vi "Actor Core.vi"(8 "error in":errorcluster, 11 "CS++DMMGui.lvclass":refnum<class "CS++DMMGui.lvclass">) -> (0 "error out":errorcluster, 3 "Actor out":refnum<class "Actor.lvclass">)   [LabVIEW 2013, in "CS++DMMGui.lvlib" / "CS++DMMGui.lvclass"]
doc: "(<B>Filename</B>: Actor Framework.lvlib:Actor.lvclass:Actor Core.vi)\n\nReceives messages to the actor, reacts to them, and initiates any error handling that may shut the actor down.\n\nDescendant classes may override this VI to append parallel tasks for the actor to complete while it handles messages. Overrides use the Call Parent Method node."
uses:
  CS++DMMGui.lvclass
  <vilib>/ActorFramework/Actor/Actor.lvclass
  Core/Actors/CS++SVMonitor/CS++SVMonitor.lvclass
  CS++DMMGui Messages/UpdateReading/UpdateReading Msg.lvclass
  CS++DMMGui Messages/UpdateMPReading/UpdateMPReading Msg.lvclass
  Core/Actors/CS++BaseActor/CS++BaseActor.lvclass/CS++BaseActor.ctl
  <vilib>/ActorFramework/Actor/Actor.lvclass/Actor.ctl
  <vilib>/ActorFramework/Message Enqueuer/Message Enqueuer.lvclass/Message Enqueuer.ctl
  Core/Actors/CS++DeviceGUIActor/CS++DeviceGUIActor.lvclass/CS++DeviceGUIActor.ctl
  Core/Classes/CS++BaseClasses/Factory/CS++Factory.lvclass
  Core/Actors/CS++PVMonitor/CS++PVMonitor.lvclass/CS++PVMonitor.ctl
  Core/Actors/CS++GUIActor/CS++GUIActor.lvclass/CS++GUIActor.ctl
  CS++DMMGui.lvclass/CS++DMMGui.ctl
  Core/Actors/CS++PVMonitor Messages/Register PVs Msg/Register PVs Msg.lvclass/Register PVs Msg.ctl
  Core/Actors/CS++DeviceGUIActor/CS++DeviceGUIActor.lvclass
  CS++DMM Messages/Configure Measurement Msg/Configure Measurement Msg.lvclass/Configure Measurement Msg.ctl
  CS++DMM Messages/Configure AC Bandwidth [AC] Msg/Configure AC Bandwidth [AC] Msg.lvclass/Configure AC Bandwidth [AC] Msg.ctl
  CS++DMM Messages/Configure Frequency Voltage Range [FVR] Msg/Configure Frequency Voltage Range [FVR] Msg.lvclass/Configure Frequency Voltage Range [FVR] Msg.ctl
  CS++DMM Messages/Configure Tranducer Type [TMP] Msg/Configure Tranducer Type [TMP] Msg.lvclass/Configure Tranducer Type [TMP] Msg.ctl
  CS++DMM Messages/Configure Thermocouple [TC] Msg/Configure Thermocouple [TC] Msg.lvclass/Configure Thermocouple [TC] Msg.ctl
  CS++DMM Messages/Configure Fixed Ref Junction [TC] Msg/Configure Fixed Ref Junction [TC] Msg.lvclass/Configure Fixed Ref Junction [TC] Msg.ctl
  CS++DMM Messages/Configure RTD [RTD] Msg/Configure RTD [RTD] Msg.lvclass/Configure RTD [RTD] Msg.ctl
  CS++DMM Messages/Configure Thermistor [THM] Msg/Configure Thermistor [THM] Msg.lvclass/Configure Thermistor [THM] Msg.ctl
  CS++DMM Messages/Configure Trigger Msg/Configure Trigger Msg.lvclass/Configure Trigger Msg.ctl
  CS++DMM Messages/Configure Trigger Slope [TS] Msg/Configure Trigger Slope [TS] Msg.lvclass/Configure Trigger Slope [TS] Msg.ctl
  CS++DMM Messages/Configure Multi-Point [MP] Msg/Configure Multi-Point [MP] Msg.lvclass/Configure Multi-Point [MP] Msg.ctl
  CS++DMM Messages/Configure Meas Complete Dest [MP] Msg/Configure Meas Complete Dest [MP] Msg.lvclass/Configure Meas Complete Dest [MP] Msg.ctl
  CS++DMM Messages/Configure Auto Zero Mode [AZ] Msg/Configure Auto Zero Mode [AZ] Msg.lvclass/Configure Auto Zero Mode [AZ] Msg.ctl
  CS++DMM Messages/Configure Power Line Frequency [PLF] Msg/Configure Power Line Frequency [PLF] Msg.lvclass/Configure Power Line Frequency [PLF] Msg.ctl
  Core/Actors/CS++DeviceGUIActor/Read Resource Name.vi
  Core/Actors/CS++DeviceGUIActor/Read Driver Revision.vi
  Core/Actors/CS++DeviceGUIActor/Read Firmware Revision.vi
  Core/Actors/CS++DeviceGUIActor/Read Self-Test Result Code.vi
  Core/Actors/CS++DeviceGUIActor/Read Self-Test Result Message.vi
  <vilib>/ActorFramework/Message Enqueuer/Init from Existing Queue.vi
  <vilib>/ActorFramework/Message Enqueuer/Enqueue.vi
  <vilib>/ActorFramework/Message Priority Queue/Priority Enqueue.vi
  <vilib>/ActorFramework/Message Enqueuer/Message Enqueuer.lvclass
  Core/Actors/CS++PVMonitor Messages/Register PVs Msg/Register PVs Msg.lvclass
  <vilib>/ActorFramework/Stop Msg/Stop Msg.lvclass
  CS++DMM Messages/Configure Measurement Msg/Configure Measurement Msg.lvclass
  CS++DMM Messages/Configure AC Bandwidth [AC] Msg/Configure AC Bandwidth [AC] Msg.lvclass
  CS++DMM Messages/Configure Frequency Voltage Range [FVR] Msg/Configure Frequency Voltage Range [FVR] Msg.lvclass
  CS++DMM Messages/Configure Tranducer Type [TMP] Msg/Configure Tranducer Type [TMP] Msg.lvclass
  CS++DMM Messages/Configure Thermocouple [TC] Msg/Configure Thermocouple [TC] Msg.lvclass
  CS++DMM Messages/Configure Fixed Ref Junction [TC] Msg/Configure Fixed Ref Junction [TC] Msg.lvclass
  CS++DMM Messages/Configure RTD [RTD] Msg/Configure RTD [RTD] Msg.lvclass
  CS++DMM Messages/Configure Thermistor [THM] Msg/Configure Thermistor [THM] Msg.lvclass
  CS++DMM Messages/Configure Trigger Msg/Configure Trigger Msg.lvclass
  CS++DMM Messages/Configure Trigger Slope [TS] Msg/Configure Trigger Slope [TS] Msg.lvclass
  CS++DMM Messages/Configure Multi-Point [MP] Msg/Configure Multi-Point [MP] Msg.lvclass
  CS++DMM Messages/Configure Meas Complete Dest [MP] Msg/Configure Meas Complete Dest [MP] Msg.lvclass
  CS++DMM Messages/Configure Auto Zero Mode [AZ] Msg/Configure Auto Zero Mode [AZ] Msg.lvclass
  CS++DMM Messages/Configure Power Line Frequency [PLF] Msg/Configure Power Line Frequency [PLF] Msg.lvclass
  Core/Actors/CS++BaseActor/CS++BaseActor.lvclass
  Core/Actors/CS++GUIActor/CS++GUIActor.lvclass
  Core/Actors/CS++PVMonitor/CS++PVMonitor.lvclass
panel:
  in  "Tab Control":T1(tab)
  out "Actor Name":string
  out "Driver Revision":string
  out "Firmware Revision":string
  out "Self-Test Result Code":i32
  out "Self-Test Result Message":string
  out "Resource Name":string
  in  "Configuration Tab":T2(tab)
  in  "freq volt range (10.0 V RMS)":dbl=10.0 format="%^.2e"
  in  "ac max frequency (300.0E+3 Hz)":dbl=300000.0 format="%^.2e"
  in  "ac min frequency (20.0 Hz)":dbl=20.0 format="%^.2e"
  in  "range (-1.0: Auto)":dbl=-1.0 format="%^.2e"
  in  "measurement function (DC Volts)":i32(ring)=1 items=["DC Volts"=1, "AC Volts"=2, "DC Current"=3, "AC Current"=4, "2 Wire Resistance"=5, "4 Wire Resistance"=101, "AC + DC Volts"=106, "AC + DC Current"=107, "Frequency"=104, "Period"=105, "Temperature"=108]
  in  "auto zero mode (Off)":i32(ring) items=["On"=1, "Off"=0, "Once"=2]
  in  "power line frequency (50.0 Hz)":dbl=50.0 caption="power line frequency (60.0 Hz)" format="%^.2e"
  in  "Tranducer Tab":enum32{"Thermocouple", "RTD", "Thermistor"}(tab)
  in  "fixed ref junc (0.0 Celsius)":dbl format="%^.2e"
  in  "ref junc type (Internal)":i32(ring)=1 items=["Internal"=1, "Fixed"=2]
  in  "thermocouple type (B)":i32(ring)=1 items=["B"=1, "C"=2, "D"=3, "E"=4, "G"=5, "J"=6, "K"=7, "N"=8, "R"=9, "S"=10, "T"=11, "U"=12, "V"=13]
  in  "resistance (0.0 ohms)":dbl format="%^.2e"
  in  "alpha (0.0)":dbl format="%^.2e"
  in  "resistance (0.0 ohms)":dbl format="%^.2e"
  in  "transducer type (Thermocouple)":i32(ring)=1 items=["Thermocouple"=1, "Thermistor"=2, "2-Wire RTD"=3, "4-Wire RTD"=4]
  in  "trigger source (Immediate)":i32(ring)=1 items=["Immediate"=1, "External"=2, "Software Trigger Function"=3, "PXI TRIG0 or VXI TTL0"=111, "PXI TRIG1 or VXI TTL1"=112, "PXI TRIG2 or VXI TTL2"=113, "PXI TRIG3 or VXI TTL3"=114, "PXI TRIG4 or VXI TTL4"=115, "PXI TRIG5 or VXI TTL5"=116, "PXI TRIG6 or VXI TTL6"=117, "PXI TRIG7 or VXI TTL7"=118, "ECL0"=119, "ECL1"=120, "PXI Star"=131, "RTSI 0"=140, "RTSI 1"=141, "RTSI 2"=142, "RTSI 3"=143, "RTSI 4"=144, "RTSI 5"=145, "RTSI 6"=146]
  in  "trigger delay (0.0 s)":dbl format="%.3f"
  in  "trigger slope (0: Positive)":i32(ring) items=["Positive", "Negative"]
  in  "sample interval (0.0 s)":dbl format="%.3f"
  in  "sample trigger (Immediate)":i32(ring)=1 items=["Immediate"=1, "External"=2, "Software Trigger Function"=3, "Interval"=10, "PXI TRIG0 or VXI TTL0"=111, "PXI TRIG1 or VXI TTL1"=112, "PXI TRIG2 or VXI TTL2"=113, "PXI TRIG3 or VXI TTL3"=114, "PXI TRIG4 or VXI TTL4"=115, "PXI TRIG5 or VXI TTL5"=116, "PXI TRIG6 or VXI TTL6"=117, "PXI TRIG7 or VXI TTL7"=118, "ECL0"=119, "ECL1"=120, "PXI Star"=131, "RTSI 0"=140, "RTSI 1"=141, "RTSI 2"=142, "RTSI 3"=143, "RTSI 4"=144, "RTSI 5"=145, "RTSI 6"=146]
  in  "trigger count (1)":i32=1
  in  "sample count (1)":i32=1
  in  "meas complete dest (None)":i32(ring)=-1 items=["None"=-1, "External"=2, "PXI TRIG0 or VXI TTL0"=111, "PXI TRIG1 or VXI TTL1"=112, "PXI TRIG2 or VXI TTL2"=113, "PXI TRIG3 or VXI TTL3"=114, "PXI TRIG4 or VXI TTL4"=115, "PXI TRIG5 or VXI TTL5"=116, "PXI TRIG6 or VXI TTL6"=117, "PXI TRIG7 or VXI TTL7"=118, "ECL0"=119, "ECL1"=120, "PXI Star"=131, "RTSI 0"=140, "RTSI 1"=141, "RTSI 2"=142, "RTSI 3"=143, "RTSI 4"=144, "RTSI 5"=145, "RTSI 6"=146]
  out "Waveform Chart":dbl(graph)
  out "Waveform Graph":dbl[](graph)
  in  "Stop Button":bool
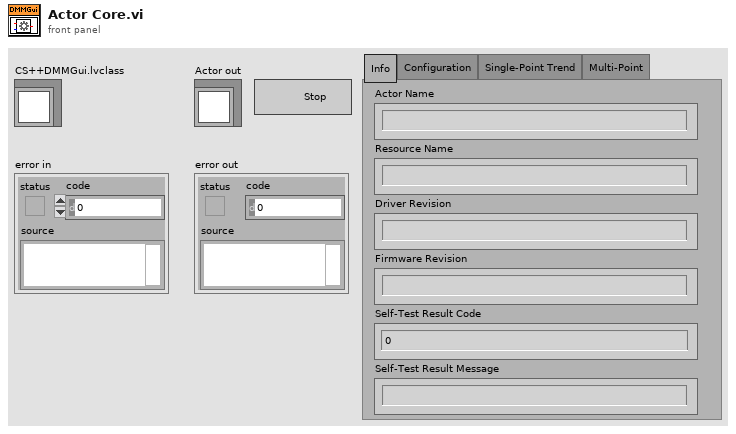
[diagram p1: front panel]
types:
  T1 = enum32{"Info", "Configuration", "Single-Point Trend", "Multi-Point"}
  T2 = enum32{"General", "Transducer", "Trigger", "Multi-Point"}
  T3 = enum32{"Invalid", "Standard", "Closed", "Hidden", "Minimized", "Maximized"}
  T4 = cluster{"name":string, "CS++DMMGui.lvlib:UpdateReading.lvclass":refnum<class "UpdateReading Msg.lvclass">}
  T5 = cluster{"name":string, "CS++DMMGui.lvlib:UpdateMPReading Msg.lvclass":refnum<class "UpdateMPReading Msg.lvclass">}
  T6 = cluster{"name":string, "CS++DMMGui.lvlib:UpdateMPReading Msg.lvclass":refnum<class "CS++PVUpdate Msg.lvclass">}[]
  T7 = cluster{"Self Enqueuer":refnum<class "Message Enqueuer.lvclass">, cluster{"name":string, "CS++DMMGui.lvlib:UpdateMPReading Msg.lvclass":refnum<class "CS++PVUpdate Msg.lvclass">}[]}
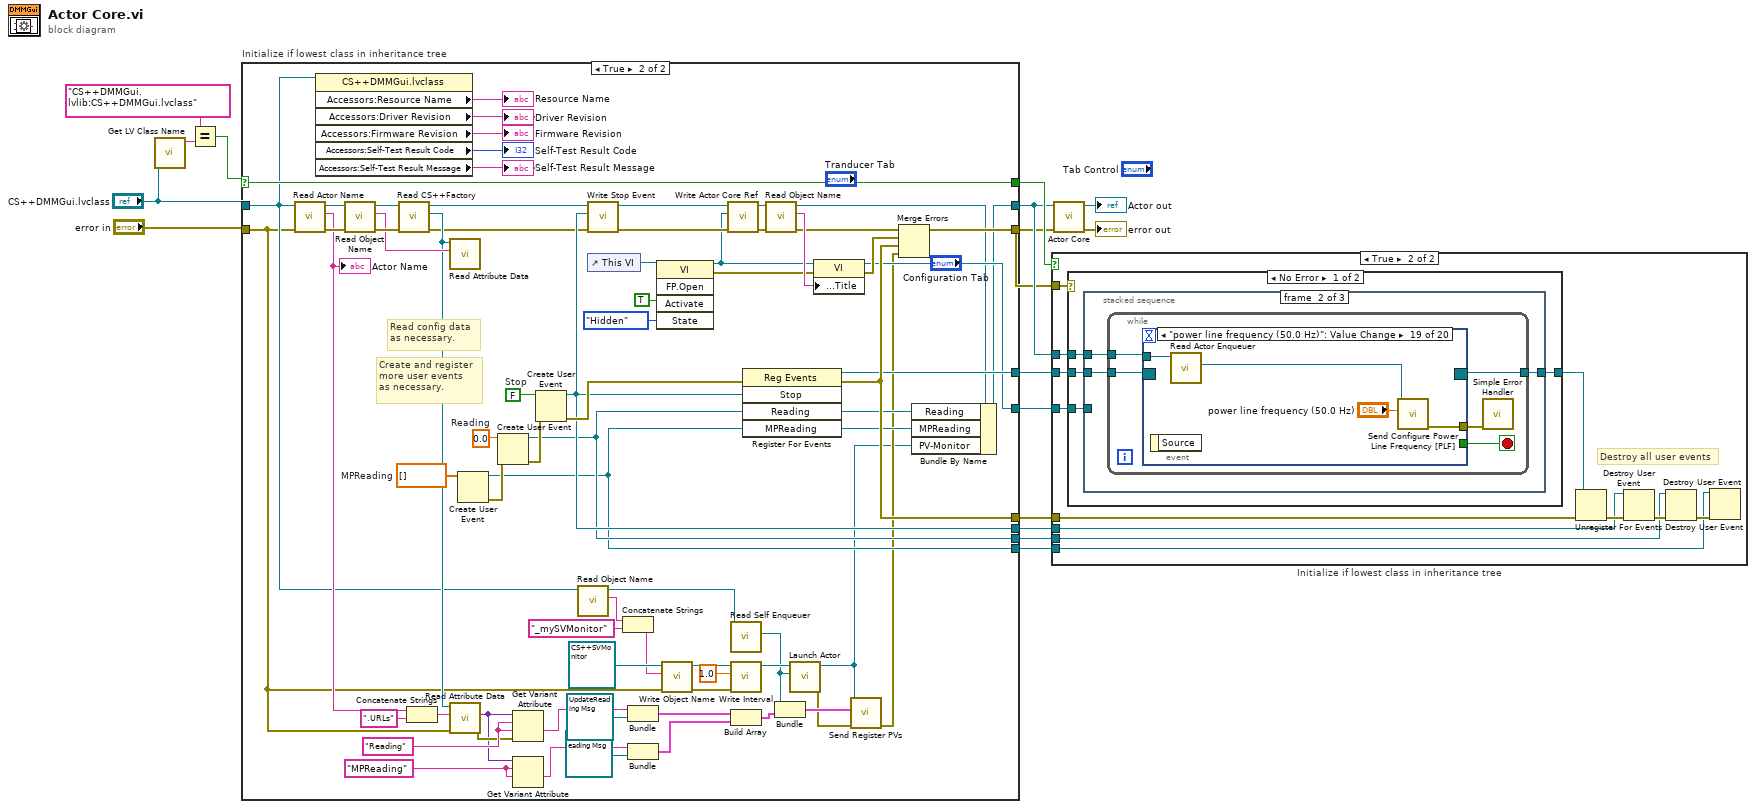
[diagram p0: block diagram]
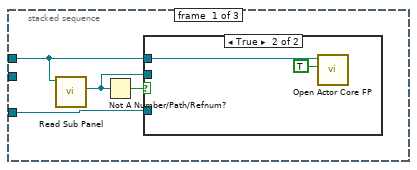
[diagram p4: hidden frame]
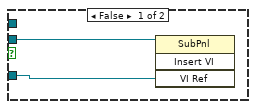
[diagram p5: hidden frame]
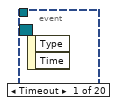
[diagram p6: hidden frame]
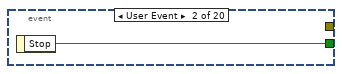
[diagram p7: hidden frame]
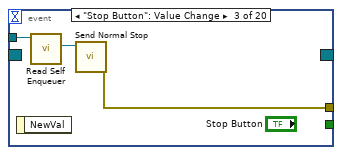
[diagram p8: hidden frame]
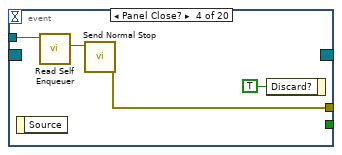
[diagram p9: hidden frame]
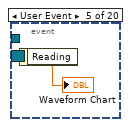
[diagram p10: hidden frame]
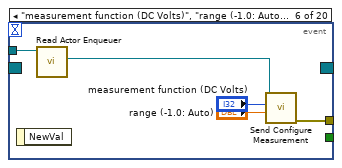
[diagram p11: hidden frame]
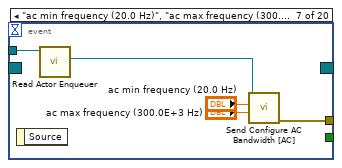
[diagram p12: hidden frame]
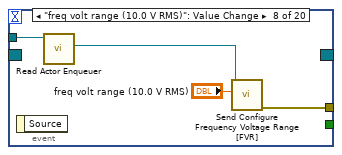
[diagram p13: hidden frame]
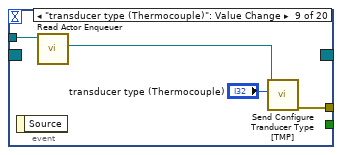
[diagram p14: hidden frame]
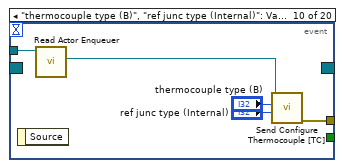
[diagram p15: hidden frame]
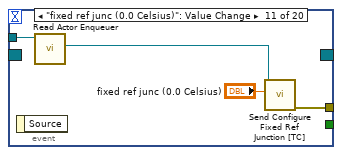
[diagram p16: hidden frame]
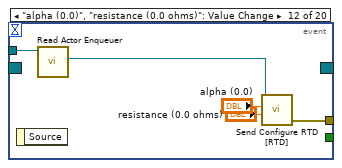
[diagram p17: hidden frame]
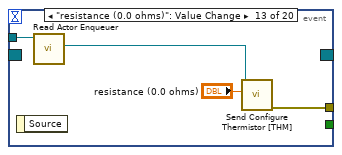
[diagram p18: hidden frame]
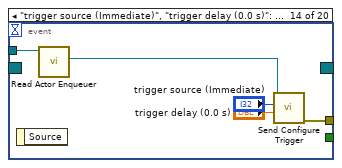
[diagram p19: hidden frame]
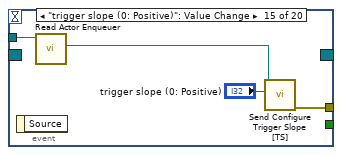
[diagram p20: hidden frame]
diagram:
  n1 = call <vilib>:"Get LV Class Name.vi"("object"="CS++DMMGui.lvclass") -> ("class name"=w14:string)  [unwired: 9 in, 1 out]
  n2 = Equal?(x="CS++DMMGui.lvlib:CS++DMMGui.lvclass" ("class name"), y=w14) -> (x = y?=w8:bool)
  n3 = case "Initialize if lowest class in inheritance tree" shown="True" w8 {
    selector: w8 -> [w17 w65]
    tunnel: [w18 w90] -> w3
    tunnel: "error in" -> [w18 w29]
    tunnel: [w19 w49] -> w4
    tunnel: "CS++DMMGui.lvclass" -> [w19 w34]
    tunnel: [_ w82] -> w12
    tunnel: [_ w81] -> w11
    tunnel: [_ w53] -> w10
    tunnel: [_ w72] -> w9
    tunnel: [w17 w65] -> w7
    tunnel: [_ w52] -> w2
    tunnel: [_ w51] -> w1
    frame False {
    }
    frame True {
      w23 = "MPReading" ("name")
      w28 = "Reading" ("name")
      w55 = dbl[] []  # MPReading
      w58 = 0.0  # Reading
      w85 = FALSE  # Stop
      # "Create and register \nmore user events\nas necessary."
      # "Read config data\nas necessary."
      n4 = call "Read Actor Name.vi"("error in (no error)"=w29, "CS++GUIActor in"=w34) -> ("error out"=w75:errorcluster, "Actor Name"=w73:string, "CS++GUIActor out"=w76:refnum<class "CS++DMMGui.lvclass">)  [unwired: 7 in]
      "Actor Name" <- w73
      n5 = property class="CS++DMMGui.lvclass"(reference=w34) -> ("Accessors:Resource Name"=→"Resource Name":string, "Accessors:Driver Revision"=→"Driver Revision":string, "Accessors:Firmware Revision"=→"Firmware Revision":string, "Accessors:Self-Test Result Code"=→"Self-Test Result Code":i32, "Accessors:Self-Test Result Message"=→"Self-Test Result Message":string)  [unwired: 1 in, 2 out]
      n6 = call "Read Object Name.vi"("error in (no error)"=w75, "CS++BaseActor in"=w76) -> ("error out"=w78:errorcluster, "Object Name"=w77:string, "CS++BaseActor out"=w79:refnum<class "CS++DMMGui.lvclass">)  [unwired: 7 in]
      n7 = call "Read CS++Factory.vi"("error in (no error)"=w78, "CS++BaseActor in"=w79) -> ("error out"=w71:errorcluster, "CS++Factory"=w74:refnum<class "CS++Factory.lvclass">, "CS++BaseActor out"=w64:refnum<class "CS++DMMGui.lvclass">)  [unwired: 7 in]
      n8 = Concatenate Strings(w73, ".URLs" ("string")) -> (w31:string)
      n9 = call-dynamic "Read Attribute Data.vi"("Object Name"=w77, "CS++Factory in"=w74) -> ()  [unwired: 7 in, 3 out]
      n10 = call-dynamic "Read Attribute Data.vi"("error in (no error)"=w29, "Object Name"=w31, "CS++Factory in"=w74) -> ("error out"=w27:errorcluster, "Attribute Data"=w24:variant)  [unwired: 6 in, 1 out]
      n11 = Create User Event(user event datatype=w55) -> (user event=w51:refnum<user-event>, error out=w56:errorcluster)  [unwired: 1 in]
      n12 = Create User Event(user event datatype=w58, error in=w56) -> (user event=w52:refnum<user-event>, error out=w57:errorcluster)
      n13 = Get Variant Attribute(Variant=w24, name=w28, default value (empty Variant)=w28, error in=w27) -> (value=w26:string)  [unwired: 3 out]
      n14 = Get Variant Attribute(Variant=w24, name=w23, default value (empty Variant)=w23) -> (value=w21:string)  [unwired: 1 in, 3 out]
      n15 = Create User Event(user event datatype=w85, error in=w57) -> (user event=w72:refnum<user-event>, error out=w83:errorcluster)
      n16 = call "Read Object Name.vi"("CS++BaseActor in"=w34) -> ("Object Name"=w41:string, "CS++BaseActor out"=w40:refnum<class "CS++DMMGui.lvclass">)  [unwired: 8 in, 1 out]
      n17 = call "Write Stop Event.vi"("error in (no error)"=w71, "Stop"=w72, "CS++GUIActor in"=w64) -> ("error out"=w69:errorcluster, "CS++GUIActor out"=w70:refnum<class "CS++DMMGui.lvclass">)  [unwired: 7 in]
      n18 = control-ref of="This VI"() -> (w89:refnum<vi>)
      n19 = Concatenate Strings(w41, "_mySVMonitor" ("Object Name")) -> (w45:string)
      n20 = Bundle("name"=w26, "CS++DMMGui.lvlib:UpdateReading.lvclass"=refnum<class "UpdateReading Msg.lvclass"> refnum) -> (w36:T4)  [unwired: 1 in]
      n21 = Bundle("name"=w21, "CS++DMMGui.lvlib:UpdateMPReading Msg.lvclass"=refnum<class "UpdateMPReading Msg.lvclass"> refnum) -> (w20:T5)  [unwired: 1 in]
      n22 = invoke class="VI" method="FP.Open"(reference=w89, "Activate"=TRUE ("Activate?"), "State"=T3."Hidden") -> (reference out=w54:refnum<vi>, error out=w80:errorcluster)  [unwired: 2 in, 3 out]
      n23 = call "Write Object Name.vi"("error in (no error)"=w29, "Object Name"=w45, "CS++BaseActor in"=refnum<class "CS++SVMonitor.lvclass"> refnum ("CS++SVMonitor.lvlib:CS++SVMonitor.lvclass")) -> ("error out"=w48:errorcluster, "CS++BaseActor out"=w46:refnum<class "CS++SVMonitor.lvclass">)  [unwired: 7 in]
      n24 = call "Write Actor Core Ref.vi"("error in (no error)"=w69, "Actor Core Ref"=w54, "CS++BaseActor in"=w70) -> ("error out"=w68:errorcluster, "CS++BaseActor out"=w67:refnum<class "CS++DMMGui.lvclass">)  [unwired: 7 in]
      n25 = call <vilib>:"Read Self Enqueuer.vi"("Actor"=w40) -> ("Self Enqueuer"=w39:refnum<class "Message Enqueuer.lvclass">)  [unwired: 10 in]
      n26 = call "Write Interval.vi"("error in (no error)"=w48, "Interval"=dbl[unit] 1.0, "CS++PVMonitor in"=w46) -> ("CS++PVMonitor out"=w44:refnum<class "CS++SVMonitor.lvclass">)  [unwired: 7 in, 1 out]
      n27 = Build Array(w36, w20) -> (w37:T6)
      n28 = register-events(error in=w83, w72, w52, w51) -> (reference out=w81:refnum<event-registration>, error out=w82:errorcluster)  [unwired: 1 in]
      n29 = call "Read Object Name.vi"("error in (no error)"=w68, "CS++BaseActor in"=w67) -> ("error out"=w66:errorcluster, "Object Name"=w86:string, "CS++BaseActor out"=w50:refnum<class "CS++DMMGui.lvclass">)  [unwired: 7 in]
      n30 = Bundle("Self Enqueuer"=w39, w37) -> (w38:T7)  [unwired: 1 in]
      n31 = call <vilib>:"Launch Actor.vi"("Actor-to-Caller Enqueuer"=w39, "Actor"=w44) -> ("error out"=w35:errorcluster, "Caller-To-Actor Enqueuer"=w32:refnum<class "Message Enqueuer.lvclass">)  [unwired: 8 in]
      n32 = property class="VI"(reference=w54, error in=w80, "Front Panel.Title"=w86) -> (reference out=w53:refnum<vi>, error out=w84:errorcluster)
      n33 = call "Send Register PVs.vi"("error in (no error)"=w35, "Register Info"=w38, "Message Enqueuer"=w32) -> ("error out"=w33:errorcluster)  [unwired: 7 in, 1 out]
      n34 = Merge Errors(w66, w84, w82, w33) -> (w90:errorcluster)
      n35 = Bundle By Name(cluster=w50, "Reading"=w52, "MPReading"=w51, "PV-Monitor"=w32) -> (w49:refnum<class "CS++DMMGui.lvclass">)
    }
  }
  n36 = case "Initialize if lowest class in inheritance tree" shown="True" w7 {
    tunnel: w3 -> [_ w102]
    tunnel: w4 -> [_ w101]
    tunnel: w12 -> [_ w99]
    tunnel: w11 -> [_ w98]
    tunnel: w10 -> [_ w96]
    tunnel: w9 -> [_ w95]
    tunnel: w2 -> [_ w92]
    tunnel: w1 -> [_ w91]
    frame False {
    }
    frame True {
      # "Destroy all user events"
      n37 = case shown="No Error" w102 {
        tunnel: w101 -> [w106 _]
        tunnel: w98 -> [w105 w199]
        tunnel: [w104 w199] -> w97
        tunnel: w96 -> [w103 _]
        frame No Error {
          n38 = stacked-sequence {
            tunnel: w106 -> [w108 w116 w198]
            tunnel: w105 -> [_ w117 _]
            tunnel: [_ w115 _] -> w104
            tunnel: w103 -> [w109 _ _]
            frame #0 {
              n39 = call "Read Sub Panel.vi"("CS++GUIActor in"=w108) -> ("Sub Panel"=w107:refnum<vi>)  [unwired: 8 in, 2 out]
              n40 = Not A Number/Path/Refnum?(number/path/refnum=w107) -> (NaN/Path/Refnum?=w110:bool)
              n41 = case shown="True" w110 {
                tunnel: w108 -> [_ w114]
                tunnel: w107 -> [w112 _]
                tunnel: w109 -> [w111 _]
                frame False {
                  n42 = invoke class="SubPnl" method="Insert VI"(reference=w112, "VI Ref"=w111) -> ()  [unwired: 2 in, 4 out]
                }
                frame True {
                  n43 = call "Open Actor Core FP.vi"("Open FP (F)"=TRUE, "CS++BaseActor in"=w114) -> ()  [unwired: 8 in, 2 out]
                }
              }
            }
            frame #1 {
              n44 = while {
                tunnel: w117 -> [w122]
                tunnel: w116 -> [w121]
                tunnel: [w119] -> w115
                stop <- w120 stop-if-true
                n45 = event shown="[18] \"power line frequency (50.0 Hz)\": Value Change" {
                  selector: w122 -> [_ _ _ _ _ _ _ _ _ _ _ _ _ _ _ _ _ _ _ _]
                  dyn-events: [_ _ _ _ _ _ _ _ _ _ _ _ _ _ _ _ _ _ _ _] -> w119
                  timeout: _ -> [_ _ _ _ _ _ _ _ _ _ _ _ _ _ _ _ _ _ _ _]
                  tunnel: w121 -> [_ _ w126 w128 _ w134 w139 w145 w149 w154 w158 w163 w166 w172 w176 w183 w187 w191 w195 _]
                  tunnel: [_ w123 _ _ _ _ _ _ _ _ _ _ _ _ _ _ _ _ _ _] -> w120
                  tunnel: [_ _ w124 w127 _ w132 w137 w142 w147 w151 w156 w160 w164 w169 w174 w178 w185 w188 w193 _] -> w118
                  event Timeout {
                    n46 = event-data() -> ()  [unwired: 1 in, 2 out]
                  }
                  event User Event {
                    n47 = event-data() -> ("Stop"=w123:bool)  [unwired: 1 in]
                  }
                  event "Stop Button": Value Change {
                    n48 = event-data() -> ()  [unwired: 1 in, 1 out]
                    n49 = call <vilib>:"Read Self Enqueuer.vi"("Actor"=w126) -> ("Self Enqueuer"=w125:refnum<class "Message Enqueuer.lvclass">)  [unwired: 10 in]
                    n50 = call <vilib>:"Send Normal Stop.vi"("Message Enqueuer"=w125) -> ("error out"=w124:errorcluster)  [unwired: 10 in]
                  }
                  event Panel Close? {
                    n51 = event-data() -> ()  [unwired: 1 in, 1 out]
                    n52 = call <vilib>:"Read Self Enqueuer.vi"("Actor"=w128) -> ("Self Enqueuer"=w129:refnum<class "Message Enqueuer.lvclass">)  [unwired: 10 in]
                    n53 = call <vilib>:"Send Normal Stop.vi"("Message Enqueuer"=w129) -> ("error out"=w127:errorcluster)  [unwired: 10 in]
                    n54 = event-data("Discard?"=TRUE) -> ()  [unwired: 1 in, 1 out]
                  }
                  event User Event {
                    n55 = event-data() -> ("Reading"=→"Waveform Chart":dbl)  [unwired: 1 in]
                  }
                  event "measurement function (DC Volts)", "range (-1.0: Auto)": Value Change {
                    n56 = event-data() -> ()  [unwired: 1 in, 1 out]
                    n57 = call "Read Actor Enqueuer.vi"("CS++GUIActor in"=w134) -> ("Actor Enqueuer"=w133:refnum<class "Message Enqueuer.lvclass">)  [unwired: 8 in, 2 out]
                    n58 = call "Send Configure Measurement.vi"("range (-1.0: Auto)"="range (-1.0: Auto)", "measurement function (DC Volts)"="measurement function (DC Volts)", "Message Enqueuer"=w133) -> ("error out"=w132:errorcluster)  [unwired: 7 in, 1 out]
                  }
                  event "ac min frequency (20.0 Hz)", "ac max frequency (300.0E+3 Hz)": Value Change {
                    n59 = event-data() -> ()  [unwired: 1 in, 1 out]
                    n60 = call "Read Actor Enqueuer.vi"("CS++GUIActor in"=w139) -> ("Actor Enqueuer"=w138:refnum<class "Message Enqueuer.lvclass">)  [unwired: 8 in, 2 out]
                    n61 = call "Send Configure AC Bandwidth [AC].vi"("ac max frequency (300.0E+3 Hz)"="ac max frequency (300.0E+3 Hz)", "ac min frequency (20.0 Hz)"="ac min frequency (20.0 Hz)", "Message Enqueuer"=w138) -> ("error out"=w137:errorcluster)  [unwired: 7 in, 1 out]
                  }
                  event "freq volt range (10.0 V RMS)": Value Change {
                    n62 = event-data() -> ()  [unwired: 1 in, 1 out]
                    n63 = call "Read Actor Enqueuer.vi"("CS++GUIActor in"=w145) -> ("Actor Enqueuer"=w143:refnum<class "Message Enqueuer.lvclass">)  [unwired: 8 in, 2 out]
                    n64 = call "Send Configure Frequency Voltage Range [FVR].vi"("freq volt range (10.0 V RMS)"="freq volt range (10.0 V RMS)", "Message Enqueuer"=w143) -> ("error out"=w142:errorcluster)  [unwired: 8 in, 1 out]
                  }
                  event "transducer type (Thermocouple)": Value Change {
                    n65 = event-data() -> ()  [unwired: 1 in, 1 out]
                    n66 = call "Read Actor Enqueuer.vi"("CS++GUIActor in"=w149) -> ("Actor Enqueuer"=w146:refnum<class "Message Enqueuer.lvclass">)  [unwired: 8 in, 2 out]
                    n67 = call "Send Configure Tranducer Type [TMP].vi"("transducer type (Thermocouple)"="transducer type (Thermocouple)", "Message Enqueuer"=w146) -> ("error out"=w147:errorcluster)  [unwired: 8 in, 1 out]
                  }
                  event "thermocouple type (B)", "ref junc type (Internal)": Value Change {
                    n68 = event-data() -> ()  [unwired: 1 in, 1 out]
                    n69 = call "Read Actor Enqueuer.vi"("CS++GUIActor in"=w154) -> ("Actor Enqueuer"=w150:refnum<class "Message Enqueuer.lvclass">)  [unwired: 8 in, 2 out]
                    n70 = call "Send Configure Thermocouple [TC].vi"("ref junc type (Internal)"="ref junc type (Internal)", "thermocouple type (B)"="thermocouple type (B)", "Message Enqueuer"=w150) -> ("error out"=w151:errorcluster)  [unwired: 7 in, 1 out]
                  }
                  event "fixed ref junc (0.0 Celsius)": Value Change {
                    n71 = event-data() -> ()  [unwired: 1 in, 1 out]
                    n72 = call "Read Actor Enqueuer.vi"("CS++GUIActor in"=w158) -> ("Actor Enqueuer"=w155:refnum<class "Message Enqueuer.lvclass">)  [unwired: 8 in, 2 out]
                    n73 = call "Send Configure Fixed Ref Junction [TC].vi"("fixed ref junc (0.0 Celsius)"="fixed ref junc (0.0 Celsius)", "Message Enqueuer"=w155) -> ("error out"=w156:errorcluster)  [unwired: 8 in, 1 out]
                  }
                  event "alpha (0.0)", "resistance (0.0 ohms)": Value Change {
                    n74 = event-data() -> ()  [unwired: 1 in, 1 out]
                    n75 = call "Read Actor Enqueuer.vi"("CS++GUIActor in"=w163) -> ("Actor Enqueuer"=w159:refnum<class "Message Enqueuer.lvclass">)  [unwired: 8 in, 2 out]
                    n76 = call "Send Configure RTD [RTD].vi"("resistance (0.0 ohms)"="resistance (0.0 ohms)", "alpha (0.0)"="alpha (0.0)", "Message Enqueuer"=w159) -> ("error out"=w160:errorcluster)  [unwired: 7 in, 1 out]
                  }
                  event "resistance (0.0 ohms)": Value Change {
                    n77 = event-data() -> ()  [unwired: 1 in, 1 out]
                    n78 = call "Read Actor Enqueuer.vi"("CS++GUIActor in"=w166) -> ("Actor Enqueuer"=w165:refnum<class "Message Enqueuer.lvclass">)  [unwired: 8 in, 2 out]
                    n79 = call "Send Configure Thermistor [THM].vi"("resistance (0.0 ohms)"="resistance (0.0 ohms)", "Message Enqueuer"=w165) -> ("error out"=w164:errorcluster)  [unwired: 8 in, 1 out]
                  }
                  event "trigger source (Immediate)", "trigger delay (0.0 s)": Value Change {
                    n80 = event-data() -> ()  [unwired: 1 in, 1 out]
                    n81 = call "Read Actor Enqueuer.vi"("CS++GUIActor in"=w172) -> ("Actor Enqueuer"=w168:refnum<class "Message Enqueuer.lvclass">)  [unwired: 8 in, 2 out]
                    n82 = call "Send Configure Trigger.vi"("trigger delay (0.0 s)"="trigger delay (0.0 s)", "trigger source (Immediate)"="trigger source (Immediate)", "Message Enqueuer"=w168) -> ("error out"=w169:errorcluster)  [unwired: 7 in, 1 out]
                  }
                  event "trigger slope (0: Positive)": Value Change {
                    n83 = event-data() -> ()  [unwired: 1 in, 1 out]
                    n84 = call "Read Actor Enqueuer.vi"("CS++GUIActor in"=w176) -> ("Actor Enqueuer"=w173:refnum<class "Message Enqueuer.lvclass">)  [unwired: 8 in, 2 out]
                    n85 = call "Send Configure Trigger Slope [TS].vi"("trigger slope (0: Positive)"="trigger slope (0: Positive)", "Message Enqueuer"=w173) -> ("error out"=w174:errorcluster)  [unwired: 8 in, 1 out]
                  }
                  event "sample interval (0.0 s)", "sample trigger (Immediate)", "trigger count (1)", "sample count (1)": Value Change {
                    n86 = event-data() -> ()  [unwired: 1 in, 1 out]
                    n87 = call "Read Actor Enqueuer.vi"("CS++GUIActor in"=w183) -> ("Actor Enqueuer"=w177:refnum<class "Message Enqueuer.lvclass">)  [unwired: 8 in, 2 out]
                    n88 = call "Send Configure Multi-Point [MP].vi"("sample count (1)"="sample count (1)", "trigger count (1)"="trigger count (1)", "sample trigger (Immediate)"="sample trigger (Immediate)", "sample interval (0.0 s)"="sample interval (0.0 s)", "Message Enqueuer"=w177) -> ("error out"=w178:errorcluster)  [unwired: 5 in, 1 out]
                  }
                  event "meas complete dest (None)": Value Change {
                    n89 = event-data() -> ()  [unwired: 1 in, 1 out]
                    n90 = call "Read Actor Enqueuer.vi"("CS++GUIActor in"=w187) -> ("Actor Enqueuer"=w184:refnum<class "Message Enqueuer.lvclass">)  [unwired: 8 in, 2 out]
                    n91 = call "Send Configure Meas Complete Dest [MP].vi"("meas complete dest (None)"="meas complete dest (None)", "Message Enqueuer"=w184) -> ("error out"=w185:errorcluster)  [unwired: 8 in, 1 out]
                  }
                  event "auto zero mode (Off)": Value Change {
                    n92 = event-data() -> ()  [unwired: 1 in, 1 out]
                    n93 = call "Read Actor Enqueuer.vi"("CS++GUIActor in"=w191) -> ("Actor Enqueuer"=w189:refnum<class "Message Enqueuer.lvclass">)  [unwired: 8 in, 2 out]
                    n94 = call "Send Configure Auto Zero Mode [AZ].vi"("auto zero mode (Off)"="auto zero mode (Off)", "Message Enqueuer"=w189) -> ("error out"=w188:errorcluster)  [unwired: 8 in, 1 out]
                  }
                  event "power line frequency (50.0 Hz)": Value Change {
                    n95 = event-data() -> ()  [unwired: 1 in, 1 out]
                    n96 = call "Read Actor Enqueuer.vi"("CS++GUIActor in"=w195) -> ("Actor Enqueuer"=w192:refnum<class "Message Enqueuer.lvclass">)  [unwired: 8 in, 2 out]
                    n97 = call "Send Configure Power Line Frequency [PLF].vi"("power line frequency (60.0 Hz)"="power line frequency (50.0 Hz)", "Message Enqueuer"=w192) -> ("error out"=w193:errorcluster)  [unwired: 8 in, 1 out]
                  }
                  event User Event {
                    n98 = event-data() -> ("MPReading"=→"Waveform Graph":dbl[])  [unwired: 1 in]
                  }
                }
                n99 = call <vilib>:"Simple Error Handler.vi"("error in (no error)"=w118) -> ()  [unwired: 4 in, 5 out]
              }
            }
            frame #2 {
              n100 = call "Open Actor Core FP.vi"("Open FP (F)"=FALSE, "CS++BaseActor in"=w198) -> ()  [unwired: 8 in, 2 out]
            }
          }
        }
        frame Error {
        }
      }
      n101 = Unregister For Events(event registration refnum=w97, error in=w99) -> (error out=w100:errorcluster)
      n102 = Destroy User Event(user event=w95, error in=w100) -> (error out=w94:errorcluster)
      n103 = Destroy User Event(user event=w92, error in=w94) -> (error out=w93:errorcluster)
      n104 = Destroy User Event(user event=w91, error in=w93) -> ()  [unwired: 1 out]
    }
  }
  n105 = call-parent "Actor Core.vi"("error in"=w3, "CS++DeviceGUIActor.lvclass"=w4) -> ("error out"=→"error out":errorcluster, "Actor out"=→"Actor out":refnum<class "Actor.lvclass">)  [unwired: 8 in]
